vi "setChannelStatus.vi"(7 "Chn":string, 8 "error in (no error)":errorcluster, 10 "State":bool, 11 "ScopeKeysight in":refnum<class "ScopeKeysight.lvclass">) -> (0 "error out":errorcluster, 3 "ScopeKeysight out":refnum<class "ScopeKeysight.lvclass">)   [LabVIEW 2023, in "ScopeKeysight.lvclass"]
doc: "<b>Author:</b> Wolfgang\n<b>Description:</b> Enable/Disable a Channel from being visible."
uses:
  ScopeKeysight.lvclass
  ScopeKeysight.lvclass/ScopeKeysight.ctl
  Driver/Keysight-DSQx3014T.lvlib
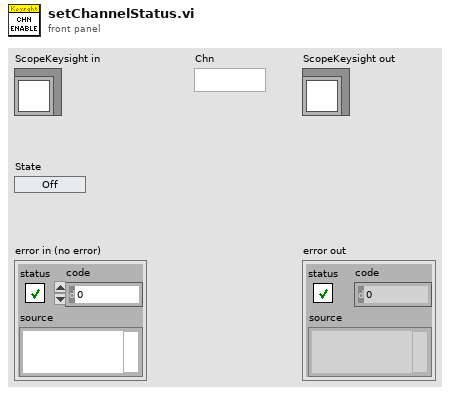
[diagram p1: front panel]
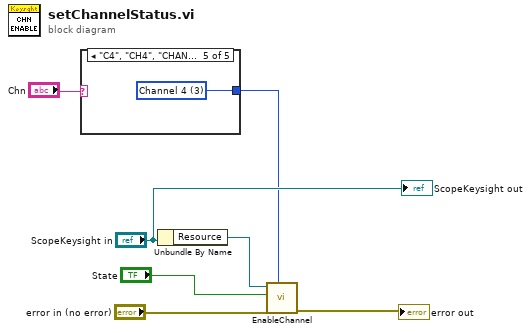
[diagram p0: block diagram]
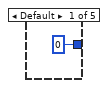
[diagram p2: hidden frame]
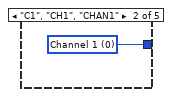
[diagram p3: hidden frame]
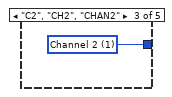
[diagram p4: hidden frame]
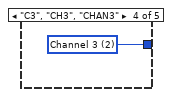
[diagram p5: hidden frame]
diagram:
  n1 = case shown="\"C4\", \"CH4\", \"CHAN4\"" "Chn" {
    tunnel: [0 ("Channel Name (0: Channel 1)") w9 w10 w11 w12] -> w1
    frame Default {
    }
    frame "C1", "CH1", "CHAN1" {
      w9 = 0 items=["Channel 1", "Channel 2", "Channel 3", "Channel 4"] ("Channel Name (0: Channel 1)")
    }
    frame "C2", "CH2", "CHAN2" {
      w10 = 1 items=["Channel 1", "Channel 2", "Channel 3", "Channel 4"] ("Channel Name (0: Channel 1)")
    }
    frame "C3", "CH3", "CHAN3" {
      w11 = 2 items=["Channel 1", "Channel 2", "Channel 3", "Channel 4"] ("Channel Name (0: Channel 1)")
    }
    frame "C4", "CH4", "CHAN4" {
      w12 = 3 items=["Channel 1", "Channel 2", "Channel 3", "Channel 4"] ("Channel Name (0: Channel 1)")
    }
  }
  n2 = Unbundle By Name("ScopeKeysight in") -> ("Resource"=w7:refnum<visa-resource-name>)
  n3 = call "EnableChannel.vi"("Channel Name (0: Channel 1)"=w1, "error in (no error)"="error in (no error)", "Enable"="State", "VISA resource name"=w7) -> ("error out"=→"error out":errorcluster)  [unwired: 6 in, 1 out]
  "ScopeKeysight out" <- "ScopeKeysight in"
